vi "DIMPowerSupply.GetTagNames.vi"(0 "i ref in":refnum<vi>, 5 "error in (no error)":errorcluster) -> (14 "i ref out":refnum<vi>, 15 "CtrTagName":string, 16 "MonTagName":string, 19 "error out":errorcluster)   [LabVIEW 2014, in "DIMPowerSupply.lvlib"]
doc: "Returns the Tag names that will be used to access the input (Monitor) and output (Control) channels of the Profibus that are connected to control and monitor the Powersupply. They are saved in Address0 and Address1 of the i-attribute."
uses:
  DIMPowerSupply.lvlib
  CSCore/BaseProcess/BaseProcess.lvlib
  CSCore/CSSystem/CSSystemLib/CSSystemLib.lvlib
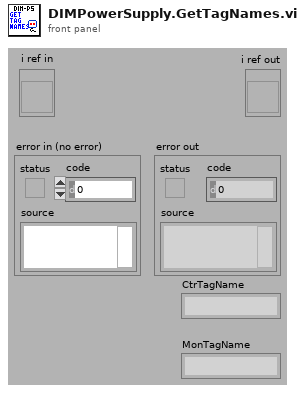
[diagram p1: front panel]
types:
  T1 = typedef "BaseProcess.lvlib/BaseProcess.i attribute.ctl" = cluster{"EventStatus":string, "EventError":i32, "PresetEvtWatchD":i32, "PresetPdcWatchD":i32, "EventTimeout":i32, "PeriodicInterval":i32, "Interface":string[], "Address":string[], "Special":string[], "PeriodicError":i32, "PeriodicStatus":string, "SuperProc":string, "Descriptors":T2[], "CaseRef":refnum<vi>, "PdcRef":refnum<vi>, "Thread Ref":refnum<vi>, "eventErrorID":i32, "eventStatusID":i32, "periodicErrorID":i32, "periodicStatusID":i32, "pdcCtrID":i32}
  T2 = typedef "BaseProcess.lvlib/BaseProcess.descriptor definition.ctl" = cluster{"selector":string, "descriptor":T3}
  T3 = typedef "BaseProcess.lvlib/BaseProcess.descriptor string definition.ctl" = string
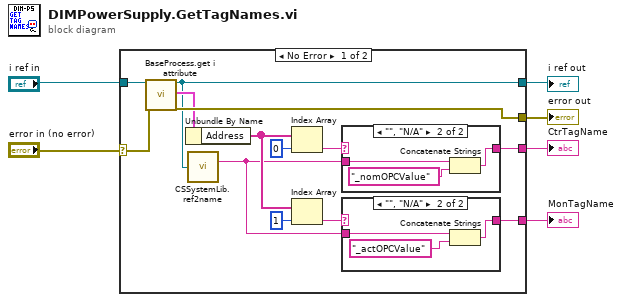
[diagram p0: block diagram]
diagram:
  n1 = case shown="No Error" "error in (no error)" {
    selector: "error in (no error)" -> [w13 w28]
    tunnel: "i ref in" -> [w19 w29]
    tunnel: [w10 w29] -> w5
    tunnel: [w18 w28] -> w4
    tunnel: [w11 _] -> w3
    tunnel: [w9 _] -> w2
    frame No Error {
      n2 = call "BaseProcess.get i attribute.vi"("i ref in"=w19, "error in (no error)"=w13) -> ("i ref out"=w10:refnum<vi>, "i attribute"=w17:T1, "error out"=w18:errorcluster)  [unwired: 15 in]
      n3 = Unbundle By Name(w17) -> ("Address"=w15:string[])
      n4 = call "CSSystemLib.ref2name.vi"("obj refnum"=w10) -> ("name"=w7:string)
      n5 = Index Array(array=w15, index=0) -> (element=w12:string)
      n6 = Index Array(array=w15, index=1) -> (element=w8:string)
      n7 = case shown="\"\", \"N/A\"" w12 {
        selector: w12 -> [w24 _]
        tunnel: [w24 w25] -> w11
        tunnel: w7 -> [_ w27]
        frame Default {
        }
        frame "", "N/A" {
          n8 = Concatenate Strings(w27, "_nomOPCValue" ("string")) -> (w25:string)
        }
      }
      n9 = case shown="\"\", \"N/A\"" w8 {
        selector: w8 -> [w20 _]
        tunnel: [w20 w21] -> w9
        tunnel: w7 -> [_ w23]
        frame Default {
        }
        frame "", "N/A" {
          n10 = Concatenate Strings(w23, "_actOPCValue" ("string")) -> (w21:string)
        }
      }
    }
    frame Error {
    }
  }
  "error out" <- w4
  "i ref out" <- w5
  "CtrTagName" <- w3
  "MonTagName" <- w2
